vi "Configure Jitter Trend.vi"(6 "Jitter Trend Vertical Span (1 %)":dbl=1.0, 7 "Jitter Trend Vertical Center (0 %)":dbl, 8 "error in (no error)":errorcluster, 9 "Jitter Trend Smoothing Points (3)":i32=3, 10 "Enable Jitter Trend Smoothing (T: Enable)":bool=TRUE, 11 "VISA resource name":refnum<visa-resource-name>) -> (0 "error out":errorcluster, 3 "VISA resource name out":refnum<visa-resource-name>)   [LabVIEW 2017, in "Agilent 2000 3000 X-Series.lvlib"]
doc: "Configures the Jitter Trend feature. Use the <b>Configure Jitter Analysis</b> VI to enable this feature.\n\n<b>Note:</b>\nThis VI is specific to the 6000-X Series oscilloscopes. These features are not available on other models."
uses:
  Agilent 2000 3000 X-Series.lvlib
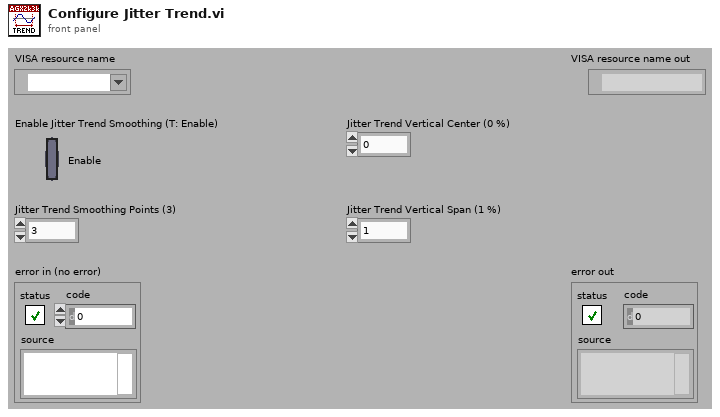
[diagram p1: front panel]
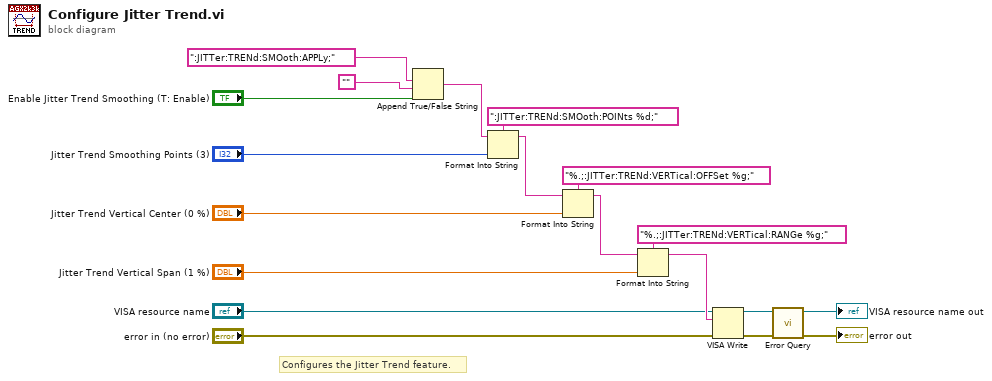
[diagram p0: block diagram]
diagram:
  # "Configures the Jitter Trend feature."
  n1 = Append True/False String(1:"Enable Jitter Trend Smoothing (T: Enable)", 2:"", 3:":JITTer:TRENd:SMOoth:APPLy;") -> (0:w6:string)  [unwired: 1 in]
  n2 = Format Into String(format string=":JITTer:TRENd:SMOoth:POINts %d;", initial string=w6, "Jitter Trend Smoothing Points (3)") -> (resulting string=w15:string)  [unwired: 1 in, 1 out]
  n3 = Format Into String(format string="%.;:JITTer:TRENd:VERTical:OFFSet %g;", initial string=w15, "Jitter Trend Vertical Center (0 %)") -> (resulting string=w12:string)  [unwired: 1 in, 1 out]
  n4 = Format Into String(format string="%.;:JITTer:TRENd:VERTical:RANGe %g;", initial string=w12, "Jitter Trend Vertical Span (1 %)") -> (resulting string=w9:string)  [unwired: 1 in, 1 out]
  n5 = VISA Write(VISA resource name="VISA resource name", write buffer=w9, error in (no error)="error in (no error)") -> (VISA resource name out=w5:refnum<visa-resource-name>, error out=w4:errorcluster)  [unwired: 1 out]
  n6 = call "Error Query.vi"("error in (no error)"=w4, "VISA resource name"=w5) -> ("error out"=→"error out":errorcluster, "VISA resource name out"=→"VISA resource name out":refnum<visa-resource-name>)  [unwired: 6 in, 2 out]
